vi "Initialize.vi"(7 "Serial Configuration":T1={"Baud Rate"=9600, "Parity"=0, "Data Bits"=8, "Stop Bits"=10, "Flow Control"=0} {"Flow Control" items=["None", "XON/XOFF", "RTS/CTS", "XON/XOFF & RTS/CTS", "DTR/DSR", "XON/XOFF & DTR/DSR"]; "Stop Bits" items=["1.0"=10, "1.5"=15, "2.0"=20]; "Data Bits" items=["7"=7, "8"=8]; "Parity" items=["None", "Odd", "Even", "Mark", "Space"]; "Baud Rate" items=["300"=300, "600"=600, "1200"=1200, "2400"=2400, "4800"=4800, "9600"=9600, "19200"=19200]}, 8 "error in":errorcluster, 9 "Reset":bool=TRUE, 10 "ID Query":bool=TRUE, 11 "VISA resource name":refnum<visa-resource-name>) -> (0 "error out":errorcluster, 3 "VISA resource name out":refnum<visa-resource-name>)   [LabVIEW 2015, in "IT-M3400.lvlib"]
doc: "Establishes communication with the instrument and optionally performs an instrument identification query and/or an instrument reset. It also places the instrument in a default state needed for other instrument driver operations. Therefore, call this VI before calling other instrument driver VIs for this instrument. Generally, you need to call the <b>Initialize</b> VI only once at the beginning of an application."
uses:
  <instrlib>/IT-M3400/IT-M3400.lvlib
panel:
  # "(c) 2014 <Enter Company Name Here>.  ALL RIGHTS RESERVED."
  # "EDIT: Change control description to remove example text for buses not supported."
  # "EDIT: Serial settings must match those on the physical instrument.  Review user's manual to determine the correct Flow Control protocol for the instrument.  \"None\" is the least robust option for this setting, and could lead to unreliable data transmission."
  # "EDIT: If your instrument does not support ID query or Reset, remove the ID Query or Reset control from the front panel and delete the case structure with the ID Query or Reset code from the block diagram."
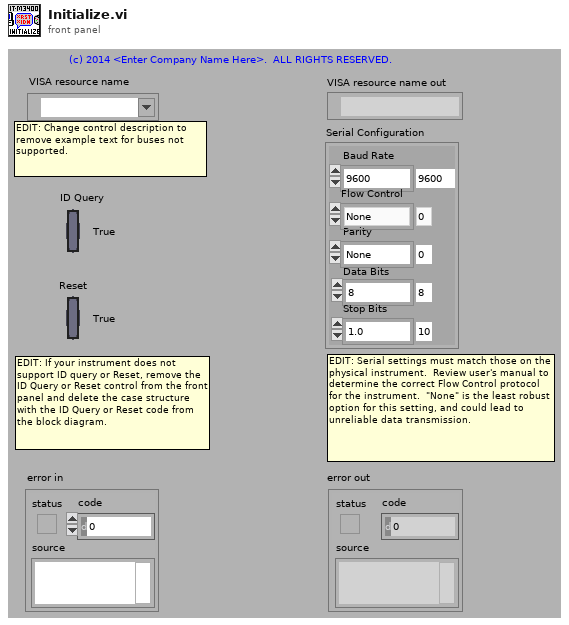
[diagram p1: front panel]
types:
  T1 = cluster{"Baud Rate":u32, "Parity":u16, "Data Bits":u16, "Stop Bits":u16, "Flow Control":u16}
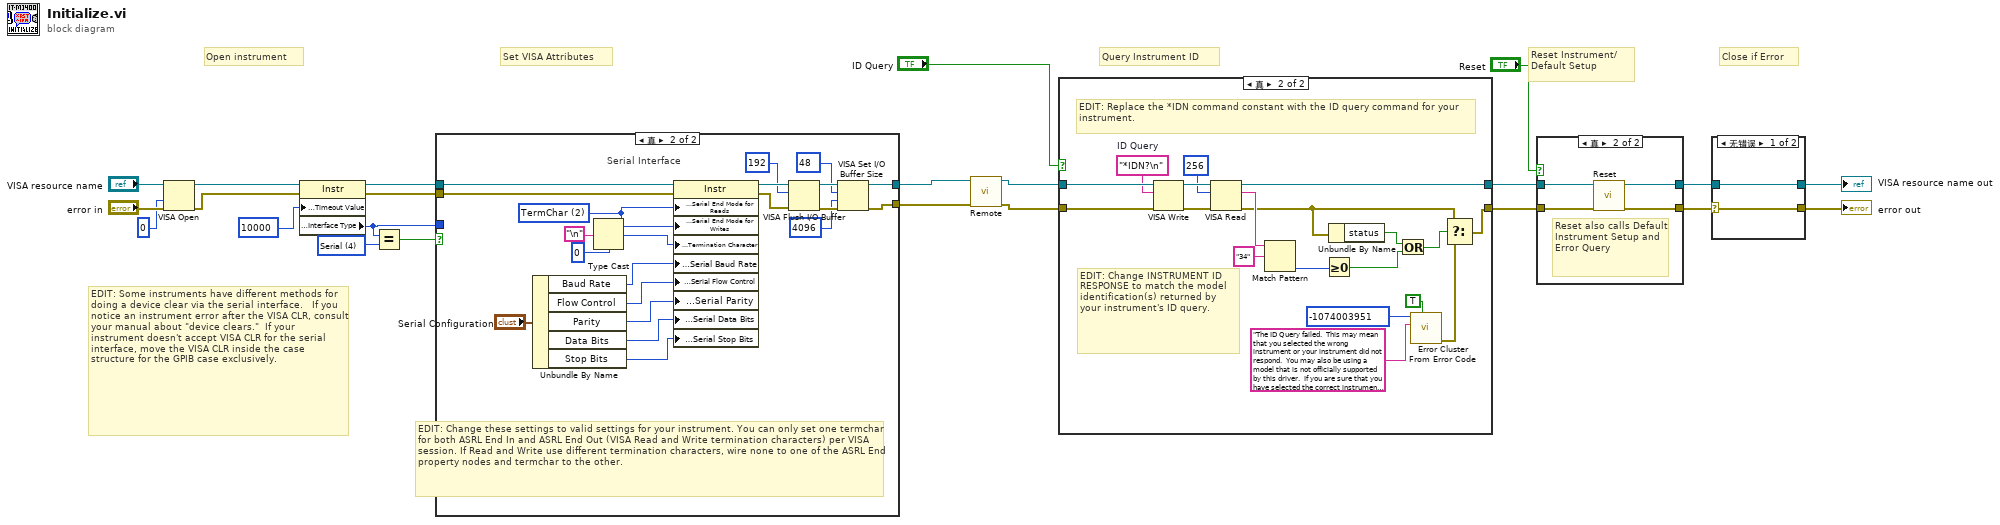
[diagram p0: block diagram]
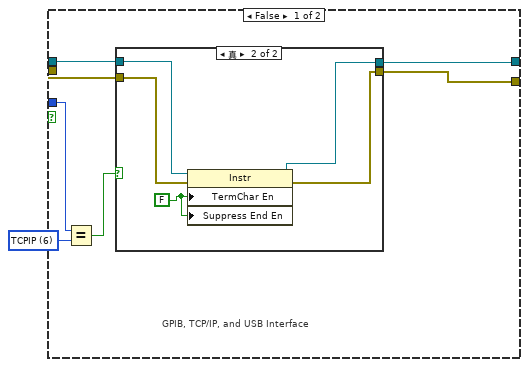
[diagram p2: hidden frame]
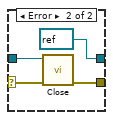
[diagram p4: hidden frame]
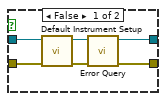
[diagram p5: hidden frame]
diagram:
  w14 = u16 4 items=["GPIB"=1, "VXI"=2, "GPIB-VXI"=3, "Serial"=4, "PXI"=5, "TCPIP"=6, "USB"=7] ("Interface Information:Interface Type")
  # "EDIT: Some instruments have different methods for doing a device clear via the serial interface.   If you notice an instrument error after the VISA CLR, consult your manual about \"device clears.\"  If your instrument doesn't accept VISA CLR for the serial interface, move the VISA CLR inside the case  structure for the GPIB case exclusively."
  # "Set VISA Attributes"
  # "Close if Error"
  # "Query Instrument ID"
  # "Reset Instrument/\nDefault Setup"
  # "Open instrument"
  n1 = VISA Open(access mode=u32 0, error in (no error)="error in", VISA resource name="VISA resource name") -> (VISA resource name=w2:refnum<visa-resource-name>, error out=w1:errorcluster)  [unwired: 2 in]
  n2 = property class="Instr"(reference=w2, error in=w1, "General Settings:Timeout Value"=u32 10000) -> (reference out=w16:refnum<visa-resource-name>, error out=w15:errorcluster, "Interface Information:Interface Type"=w8:u16)
  n3 = Equal?(x=w8, y=w14) -> (x = y?=w3:bool)
  n4 = case shown="真" w3 {
    tunnel: [w25 w55] -> w7
    tunnel: [w24 w52] -> w6
    tunnel: w16 -> [w27 w57]
    tunnel: w15 -> [w26 w58]
    tunnel: w8 -> [w28 _]
    frame False {
      w29 = u16 6 items=["GPIB"=1, "VXI"=2, "GPIB-VXI"=3, "Serial"=4, "PXI"=5, "TCPIP"=6, "USB"=7] ("Interface Information:Interface Type")
      # "GPIB, TCP/IP, and USB Interface"
      n5 = Equal?(x=w28, y=w29) -> (x = y?=w30:bool)
      n6 = case shown="真" w30 {
        tunnel: [w32 w37] -> w25
        tunnel: [w31 w36] -> w24
        tunnel: w27 -> [w32 w34]
        tunnel: w26 -> [w31 w33]
        frame False {
        }
        frame True {
          w35 = FALSE
          n7 = property class="Instr"(reference=w34, error in=w33, "TermChar En"=w35, "Suppress End En"=w35) -> (reference out=w37:refnum<visa-resource-name>, error out=w36:errorcluster)
        }
      }
    }
    frame True {
      w45 = u16 2 items=["None", "LastBit", "TermChar"] ("Serial Settings:Serial End Mode for Reads")
      # "EDIT: Change these settings to valid settings for your instrument. You can only set one termchar for both ASRL End In and ASRL End Out (VISA Read and Write termination characters) per VISA session. If Read and Write use different termination characters, wire none to one of the ASRL End property nodes and termchar to the other."
      # "Serial Interface"
      n8 = Unbundle By Name("Serial Configuration") -> ("Baud Rate"=w43:u32, "Flow Control"=w39:u16, "Parity"=w41:u16, "Data Bits"=w42:u16, "Stop Bits"=w38:u16)
      n9 = Type Cast(type=u8 0, x="\n" ("Line Feed Constant")) -> (*(type *) &x=w44:u8)
      n10 = property class="Instr"(reference=w57, error in=w58, "Serial Settings:Serial End Mode for Reads"=w45, "Serial Settings:Serial End Mode for Writes"=w45, "Message Based Settings:Termination Character"=w44, "Serial Settings:Serial Baud Rate"=w43, "Serial Settings:Serial Flow Control"=w39, "Serial Settings:Serial Parity"=w41, "Serial Settings:Serial Data Bits"=w42, "Serial Settings:Serial Stop Bits"=w38) -> (reference out=w51:refnum<visa-resource-name>, error out=w54:errorcluster)
      n11 = VISA Flush I/O Buffer(VISA resource name=w51, mask (16)=u16 192, error in (no error)=w54) -> (VISA resource name out=w56:refnum<visa-resource-name>, error out=w53:errorcluster)
      n12 = VISA Set I/O Buffer Size(VISA resource name=w56, mask (16)=u16 48, size (4096)=u32 4096 ("size (0)"), error in (no error)=w53) -> (VISA resource name out=w55:refnum<visa-resource-name>, error out=w52:errorcluster)
    }
  }
  n13 = call <instrlib>:"Remote.vi"("error in"=w6, "VISA resource name"=w7) -> ("error out"=w4:errorcluster, "VISA resource name out"=w5:refnum<visa-resource-name>)  [unwired: 8 in]
  n14 = case shown="真" "ID Query" {
    tunnel: [w59 w79] -> w22
    tunnel: [w60 w76] -> w23
    tunnel: w5 -> [w60 w77]
    tunnel: w4 -> [w59 w78]
    frame False {
    }
    frame True {
      w70 = "*IDN?\n"  # ID Query
      # "EDIT: Replace the *IDN command constant with the ID query command for your instrument."
      # "EDIT: Change INSTRUMENT ID RESPONSE to match the model identification(s) returned by your instrument's ID query."
      n15 = VISA Write(VISA resource name=w77, write buffer=w70, error in (no error)=w78) -> (VISA resource name out=w74:refnum<visa-resource-name>, error out=w73:errorcluster)  [unwired: 1 out]
      n16 = VISA Read(VISA resource name=w74, byte count=u32 256, error in (no error)=w73) -> (VISA resource name out=w76:refnum<visa-resource-name>, read buffer=w75:string, error out=w64:errorcluster)  [unwired: 1 out]
      n17 = Match Pattern(string=w75, regular expression="34") -> (offset past match=w65:i32)  [unwired: 1 in, 3 out]
      n18 = Greater Or Equal To 0?(x=w65) -> (x >= 0?=w62:bool)
      n19 = Unbundle By Name(w64) -> ("status"=w63:bool)
      n20 = Or(x=w63, y=w62) -> (x .or. y?=w61:bool)
      n21 = call <vilib>:"Error Cluster From Error Code.vi"("show call chain? (False)"=TRUE, "error message (\"\")"="The ID Query failed.  This may mean that you selected the wrong instrument or your instrument did not respond.  You may also be using a model that is not officially supported by this driver.  If you are sure that you have selected the correct instrument and it is responding, try disabling the ID Query." ("Source (VI Name)"), "error code (0)"=-1074003951 ("Code")) -> ("error out"=w69:errorcluster)  [unwired: 6 in]
      n22 = Select(t=w64, s=w61, f=w69) -> (s? t:f=w79:errorcluster)
    }
  }
  n23 = case shown="真" "Reset" {
    tunnel: w22 -> [w84 w86]
    tunnel: [w81 w89] -> w9
    tunnel: w23 -> [w85 w87]
    tunnel: [w82 w88] -> w10
    frame False {
      n24 = call <instrlib>:"Default Instrument Setup.vi"("error in"=w84, "VISA resource name"=w85) -> ("error out"=w80:errorcluster, "VISA resource name out"=w83:refnum<visa-resource-name>)  [unwired: 8 in]
      n25 = call <instrlib>:"Error Query.vi"("error in"=w80, "VISA resource name"=w83) -> ("error out"=w81:errorcluster, "VISA resource name out"=w82:refnum<visa-resource-name>)  [unwired: 6 in, 2 out]
    }
    frame True {
      # "Reset also calls Default Instrument Setup and Error Query"
      n26 = call <instrlib>:"Reset.vi"("error in"=w86, "VISA resource name"=w87) -> ("error out"=w89:errorcluster, "VISA resource name out"=w88:refnum<visa-resource-name>)  [unwired: 8 in]
    }
  }
  n27 = case shown="无错误" w9 {
    selector: w9 -> [w90 w93]
    tunnel: w10 -> [w91 w94]
    tunnel: [w91 refnum<visa-resource-name> refnum ("VISA resource name out")] -> w12
    tunnel: [w90 w95] -> w11
    frame No Error {
    }
    frame Error {
      n28 = call <instrlib>:"Close.vi"("error in"=w93, "VISA resource name"=w94) -> ("error out"=w95:errorcluster)  [unwired: 9 in]
    }
  }
  "VISA resource name out" <- w12
  "error out" <- w11
